vi "NIIE_Tree Set All.vi"(8 "Error":errorcluster, 10 "Value":string, 11 "TreeControl":refnum<vi>) -> (0 "Error Out":errorcluster, 3 "TreeControl Out":refnum<vi>)   [LabVIEW 2021]
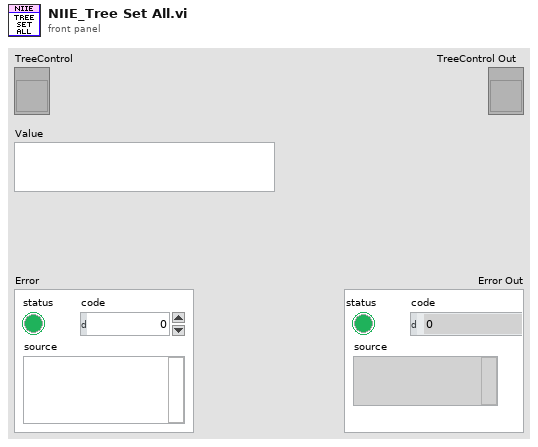
[diagram p1: front panel]
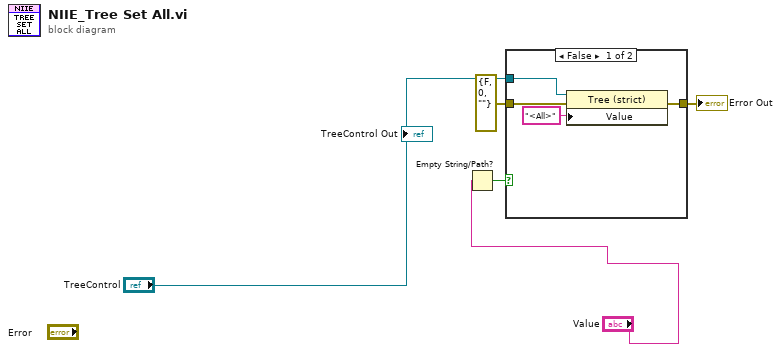
[diagram p0: block diagram]
diagram:
  n1 = Empty String/Path?(string/path="Value") -> (empty?=w1:bool)
  n2 = case shown="False" w1 {
    tunnel: errorcluster {"status"=FALSE, "code"=0, "source"=""} ("error out") -> [w7 w10]
    tunnel: [w9 w10] -> w5
    tunnel: "TreeControl" -> [w8 _]
    frame False {
      n3 = property class="Tree (strict)"(reference=w8, error in=w7, "Value"="<All>") -> (error out=w9:errorcluster)  [unwired: 1 out]
    }
    frame True {
    }
  }
  "Error Out" <- w5
